vi "RestartSensor.vi"(8 "error in (no error)":errorcluster, 9 "milliseconds to wait":u32=1000, 10 "Address":u8, 11 "VISA resource name":refnum<visa-resource-name>) -> (0 "error out":errorcluster, 3 "VISA resource name out":refnum<visa-resource-name>)   [LabVIEW 2020, in "driver_flodx_rtd.lvlib"]
doc: "Restarts the device"
uses:
  <instrlib>/RxnRover/FloDx RTD Driver/driver_flodx_rtd.lvlib
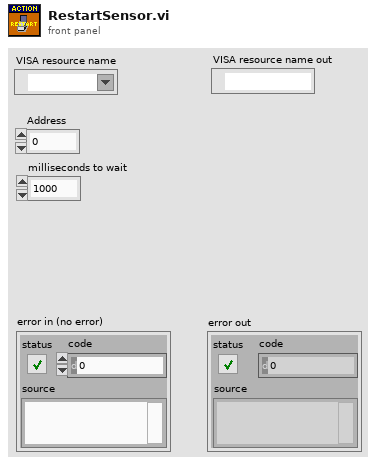
[diagram p1: front panel]
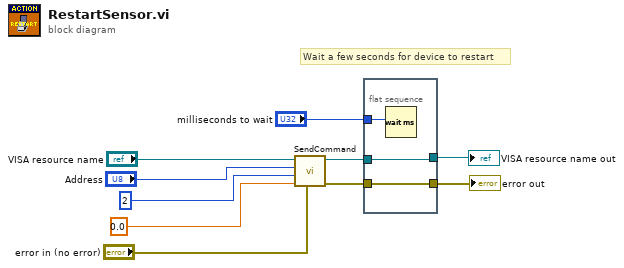
[diagram p0: block diagram]
diagram:
  # "Wait a few seconds for device to restart"
  n1 = call <instrlib>:"SendCommand.vi"("error in"="error in (no error)", "Parameter"=sgl 0.0, "Command"=u8 2, "Address"="Address", "VISA resource name"="VISA resource name") -> ("error out"=w4:errorcluster, "VISA resource name out"=w3:refnum<visa-resource-name>)  [unwired: 4 in, 1 out]
  n2 = flat-sequence {
    tunnel: [w13] -> w5
    tunnel: w4 -> [w13]
    tunnel: [w12] -> w2
    tunnel: w3 -> [w12]
    tunnel: "milliseconds to wait" -> [w11]
    frame #0 {
      n3 = Wait (ms)(milliseconds to wait=w11) -> ()  [unwired: 1 out]
    }
  }
  "VISA resource name out" <- w2
  "error out" <- w5
